vi "LakeShore218_input_onoff.vi"(8 "error in":errorcluster, 9 "onoff":enum16{"Off", "On"}(ring), 10 "channel":i8=1, 11 "VISA in":refnum<visa-resource-name>) -> (0 "error out":errorcluster, 3 "VISA out":refnum<visa-resource-name>, 4 "status":bool)   [LabVIEW 2019]
panel:
  out "string":string
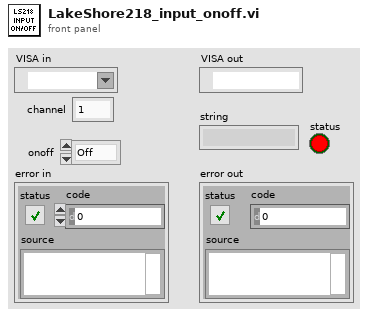
[diagram p1: front panel]
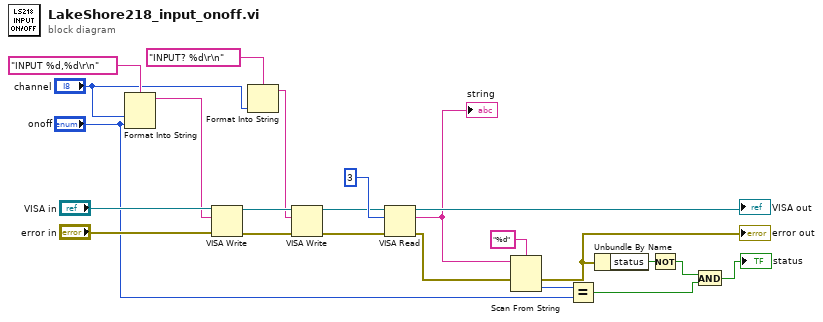
[diagram p0: block diagram]
diagram:
  n1 = Format Into String(format string="INPUT %d,%d\r\n", "channel", "onoff") -> (resulting string=w13:string)  [unwired: 2 in, 1 out]
  n2 = VISA Write(VISA resource name="VISA in", write buffer=w13, error in (no error)="error in") -> (VISA resource name out=w8:refnum<visa-resource-name>, error out=w10:errorcluster)  [unwired: 1 out]
  n3 = Format Into String(format string="INPUT? %d\r\n", "channel") -> (resulting string=w6:string)  [unwired: 2 in, 1 out]
  n4 = VISA Write(VISA resource name=w8, write buffer=w6, error in (no error)=w10) -> (VISA resource name out=w7:refnum<visa-resource-name>, error out=w9:errorcluster)  [unwired: 1 out]
  n5 = VISA Read(VISA resource name=w7, byte count=u32 3, error in (no error)=w9) -> (VISA resource name out=→"VISA out":refnum<visa-resource-name>, read buffer=w19:string, error out=w17:errorcluster)  [unwired: 1 out]
  "string" <- w19
  n6 = Scan From String(format string="%d", input string=w19, error in=w17) -> (error out=w16:errorcluster, output 1=w5:i32)  [unwired: 2 in, 2 out]
  "error out" <- w16
  n7 = Equal?(x=w5, y="onoff") -> (x = y?=w1:bool)
  n8 = Unbundle By Name(w16) -> ("status"=w15:bool)
  n9 = Not(x=w15) -> (.not. x?=w2:bool)
  n10 = And(x=w2, y=w1) -> (x .and. y?=→"status":bool)
